vi "Choose_Plug_In_to_Run.vi"(2 "setup":T1, 3 "Show Panel?":bool, 4 "Setup String In":string) -> (1 "Setup String Out":string)   [LabVIEW 2022 SP3]
uses:
  Anemometry Sub Vis/Controls/ok_button.ctl
  Anemometry Sub Vis/Controls/Setup.ctl
  Anemometry Sub Vis/Controls/Post_Process.ctl
  Anemometry Sub Vis/Globals/Meas_global.vi
  Anemometry Sub Vis/Globals/Dynamic_call_global.ph.vi
panel:
  in  "Deselect Pre Analysis Plugins":bool
  in  "Pre_Analysis_Plugins":i32[](listbox)
  in  "Deselect Final":bool
  in  "Deselect per block":bool
  in  "Deselect Initial":bool
  in  "Override Post Process Plugins Setup":bool
  in  "OK Button":T2
  in  "Final Plug In":i32[](listbox)
  in  "Per Block Plug ins":i32[](listbox)
  in  "Initial Plug Ins":i32[](listbox)
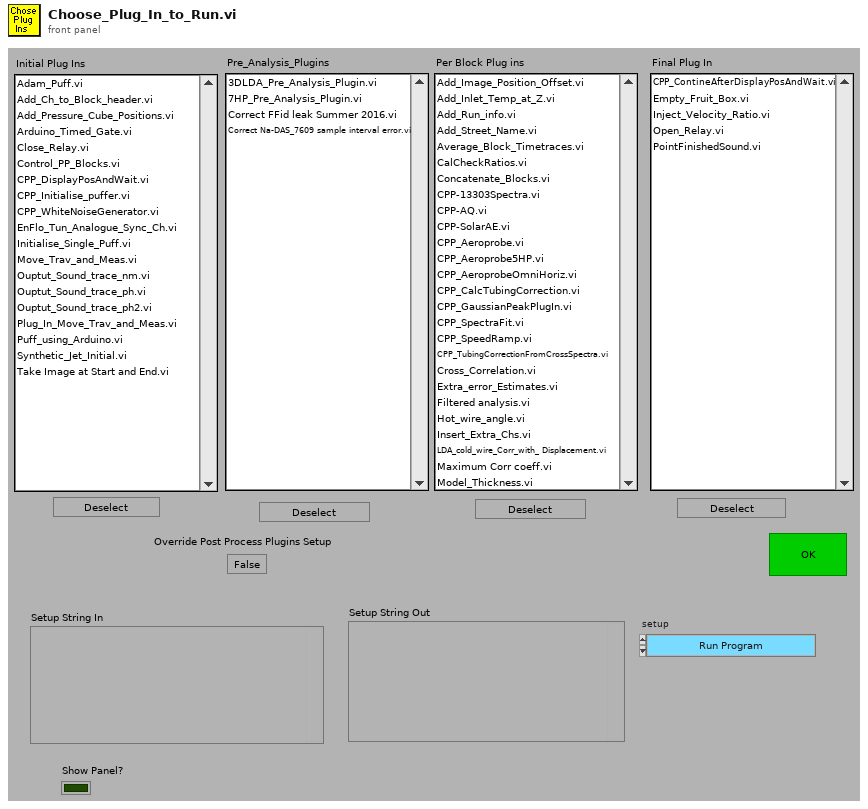
[diagram p1: front panel]
types:
  T1 = typedef "Setup.ctl" = enum16{"Run Program", "Show Setup", "Save Current Setup", "Setup Front Panel"}
  T2 = typedef "ok_button.ctl" = bool
  T3 = typedef "Post_Process.ctl" = enum16{"Take New Data", "Post Process Raw Data File"}
  T4 = enum32{"Invalid", "Standard", "Closed", "Hidden", "Minimized", "Maximized"}
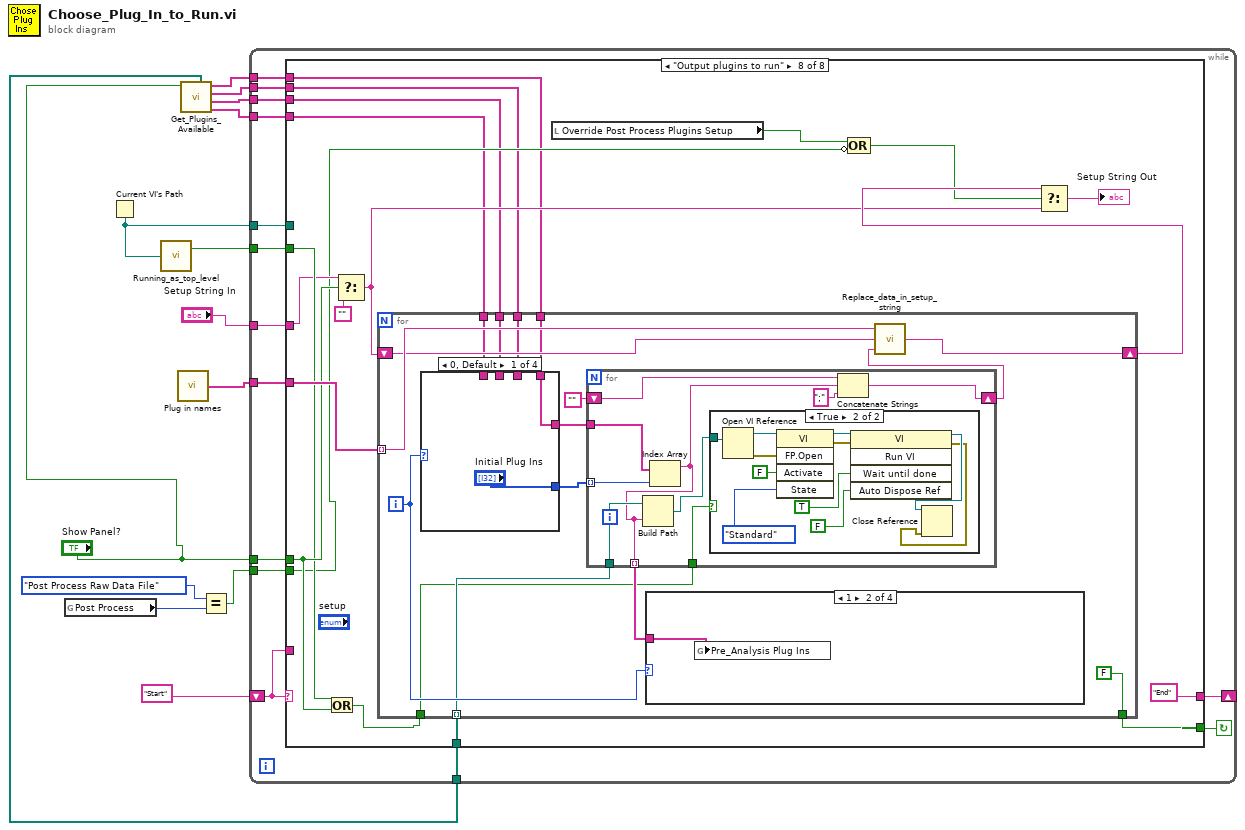
[diagram p0: block diagram]
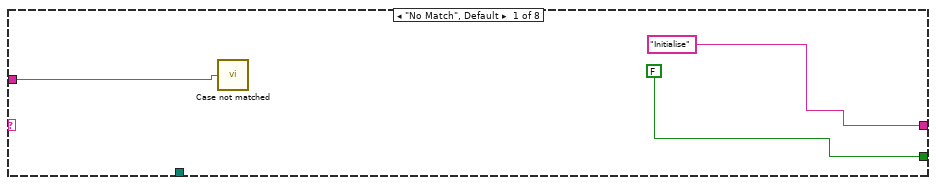
[diagram p2: hidden frame]
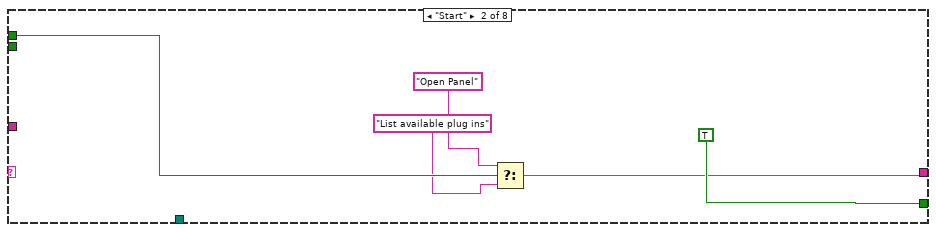
[diagram p3: hidden frame]
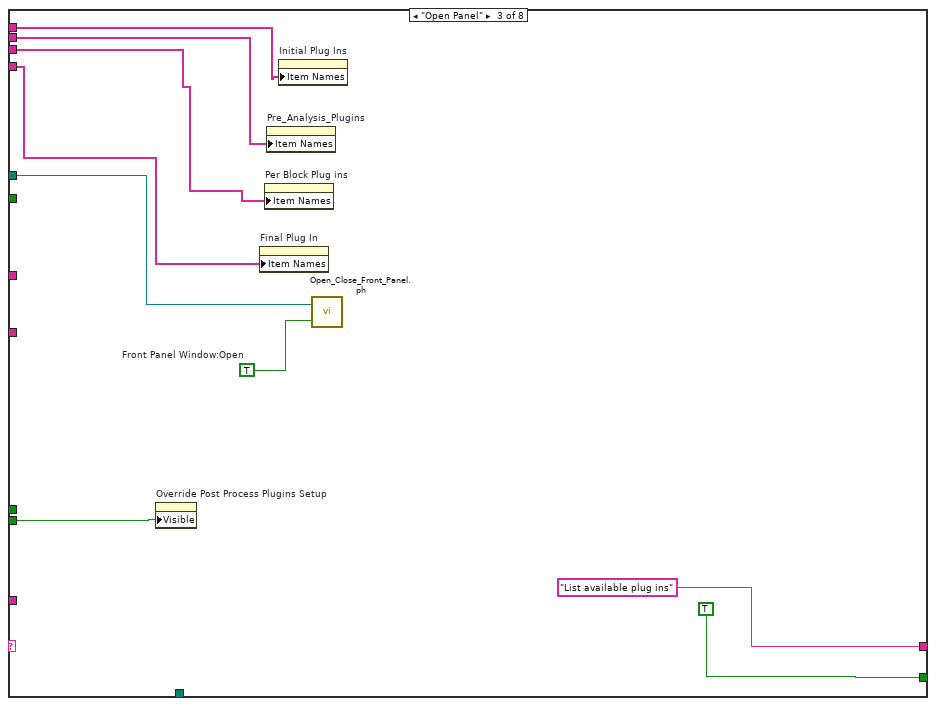
[diagram p4: hidden frame]
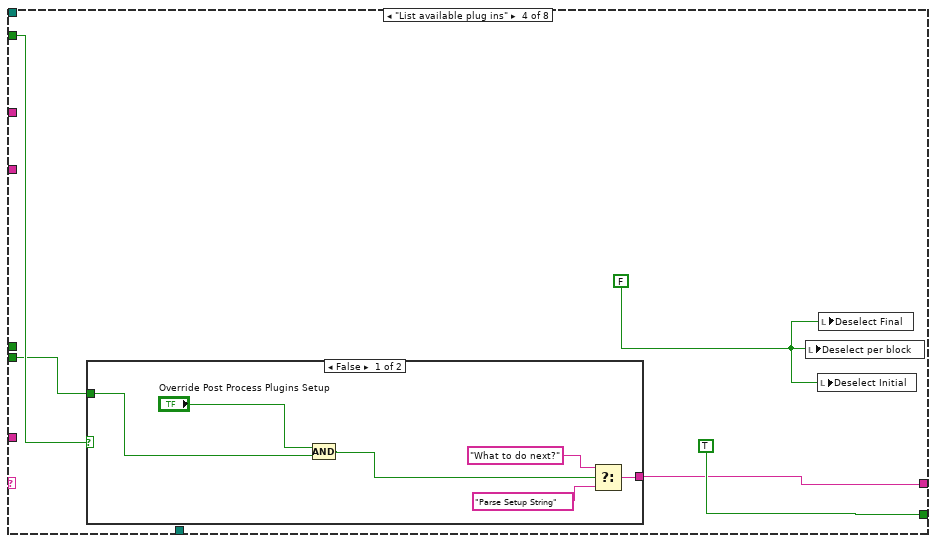
[diagram p5: hidden frame]
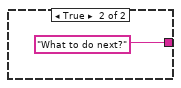
[diagram p6: hidden frame]
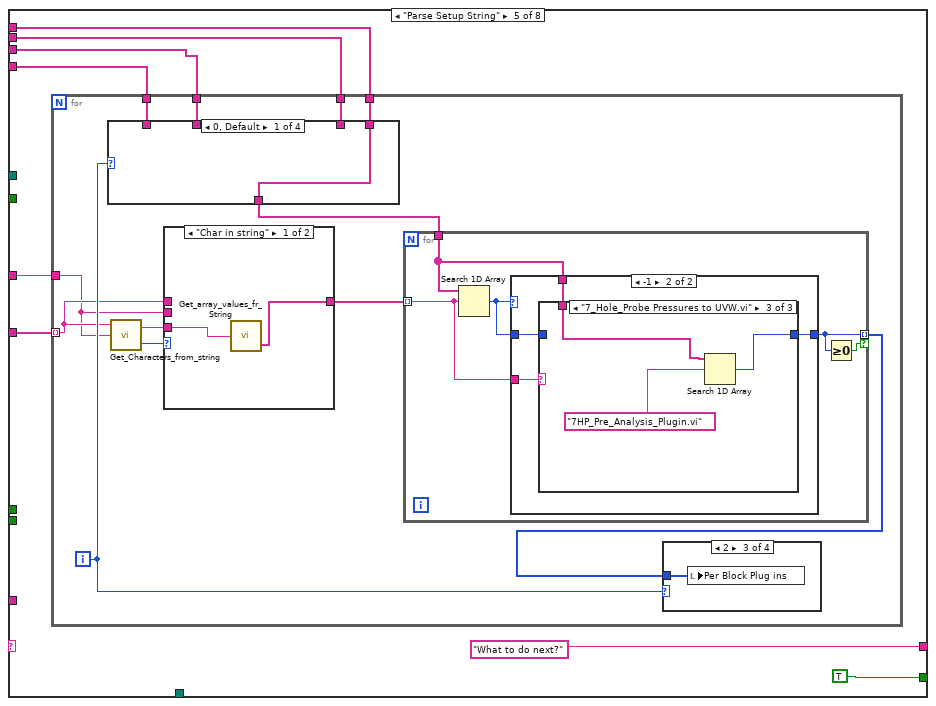
[diagram p7: hidden frame]
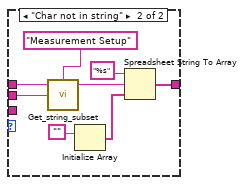
[diagram p8: hidden frame]
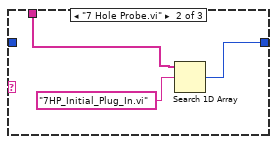
[diagram p11: hidden frame]
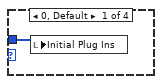
[diagram p15: hidden frame]
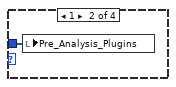
[diagram p16: hidden frame]
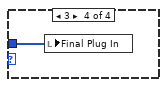
[diagram p17: hidden frame]
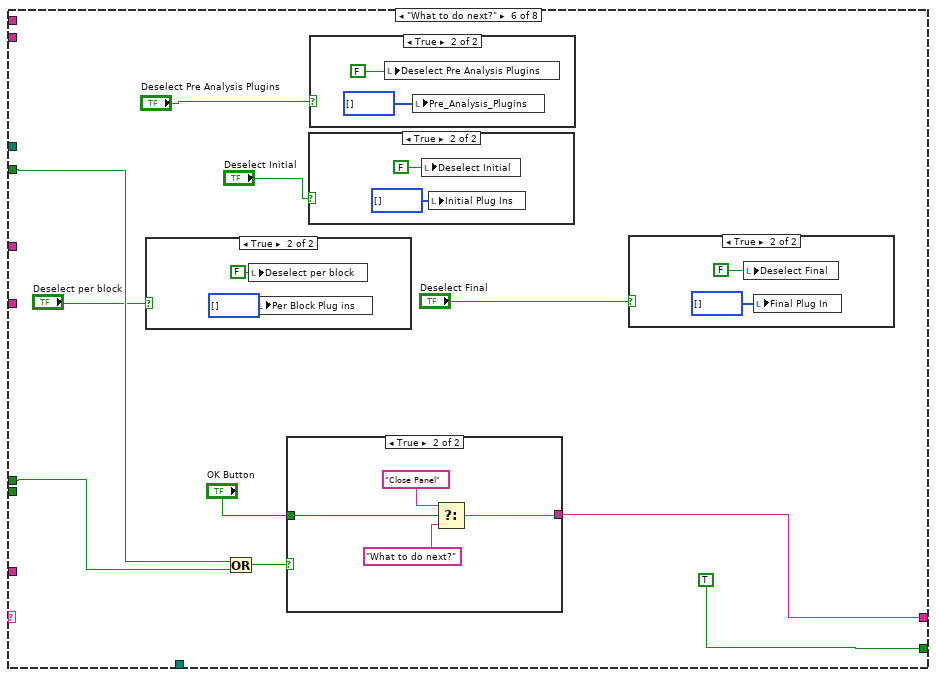
[diagram p18: hidden frame]
diagram:
  n1 = global read "Meas_global.vi" "Post Process"() -> (w9:T3)
  n2 = Current VI's Path() -> (path=w11:path)
  n3 = call "Running_as_top_level.vi"("Vi path name"=w11) -> ("Top Level"=w12:bool)  [unwired: 1 out]
  n4 = call "Plug in names.vi"() -> ("Array"=w1:string[])  [unwired: 1 in]
  n5 = call "Get_Plugins_Available.vi"("Reload Available Plugins"="Show Panel?") -> ("Final"=w4:string[], "Per Block"=w5:string[], "Pre-Analysis"=w6:string[], "Initial"=w7:string[], "Directories"=w3:path[])  [unwired: 6 in]
  n6 = Equal?(x=Post_Process."Post Process Raw Data File" ("Post Process"), y=w9) -> (x = y?=w8:bool)
  n7 = while {
    shift-left: "Start" -> [w26]
    shift-right: [w27] -> _
    tunnel: w1 -> [w25]
    tunnel: "Show Panel?" -> [w24]
    tunnel: "Setup String In" -> [w23]
    tunnel: w12 -> [w22]
    tunnel: w11 -> [w21]
    tunnel: w8 -> [w20]
    tunnel: w7 -> [w19]
    tunnel: w6 -> [w18]
    tunnel: w5 -> [w17]
    tunnel: w4 -> [w16]
    tunnel: w3 -> [w15]
    stop <- w28 continue-if-true
    n8 = case shown="\"Output plugins to run\"" w26 {
      tunnel: [FALSE TRUE TRUE TRUE TRUE TRUE TRUE w151] -> w28
      tunnel: ["Initialise" w32 "List available plug ins" ("f") w49 "What to do next?" ("t") w120 "Output plugins to run" ("f") "End"] -> w27
      tunnel: w26 -> [w29 _ _ _ _ _ _ _]
      tunnel: w25 -> [_ _ _ _ w64 _ _ w169]
      tunnel: w24 -> [_ w34 _ _ _ w119 _ w167]
      tunnel: w23 -> [_ _ _ _ w63 _ _ w161]
      tunnel: w22 -> [_ _ _ w48 _ w118 w138 w166]
      tunnel: w21 -> [_ _ w42 _ _ _ _ _]
      tunnel: w20 -> [_ _ w41 w46 _ _ w136 w157]
      tunnel: w19 -> [_ _ w37 _ w61 _ _ w156]
      tunnel: w18 -> [_ _ w38 _ w60 _ _ w155]
      tunnel: w17 -> [_ _ w39 _ w59 _ _ w154]
      tunnel: w16 -> [_ _ w40 _ w58 _ _ w153]
      tunnel: w15 -> [_ _ _ _ _ _ _ w152]
      frame "No Match", Default {
        n9 = call "Case not matched.vi"("Case Name not Matched"=w29) -> ()
      }
      frame "Start" {
        n10 = Select(t="Open Panel", s=w34, f="List available plug ins") -> (s? t:f=w32:string)
      }
      frame "Open Panel" {
        w44 = TRUE  # Front Panel Window:Open
        n11 = property on="Override Post Process Plugins Setup" class="Bool (strict)"("Visible"=w41) -> ()  [unwired: 2 in, 2 out]
        n12 = property on="Final Plug In" class="LstBox (strict)"("Item Names"=w40) -> ()  [unwired: 2 in, 2 out]
        n13 = property on="Per Block Plug ins" class="LstBox (strict)"("Item Names"=w39) -> ()  [unwired: 2 in, 2 out]
        n14 = property on="Pre_Analysis_Plugins" class="LstBox (strict)"("Item Names"=w38) -> ()  [unwired: 2 in, 2 out]
        n15 = property on="Initial Plug Ins" class="LstBox (strict)"("Item Names"=w37) -> ()  [unwired: 2 in, 2 out]
        n16 = call "Open_Close_Front_Panel.ph.vi"("openWindow (T)"=w44, "VI path"=w42) -> ()  [unwired: 1 in, 1 out]
      }
      frame "List available plug ins" {
        w47 = FALSE
        n17 = case shown="False" w48 {
          tunnel: [w52 "What to do next?"] -> w49
          tunnel: w46 -> [w51 _]
          frame False {
            n18 = Compound Arithmetic op=AND("Override Post Process Plugins Setup", w51) -> (w55:bool)
            n19 = Select(t="What to do next?", s=w55, f="Parse Setup String") -> (s? t:f=w52:string)
          }
          frame True {
          }
        }
        n20 = local write "Deselect per block"(w47) -> ()
        n21 = local write "Deselect Initial"(w47) -> ()
        n22 = local write "Deselect Final"(w47) -> ()
      }
      frame "Parse Setup String" {
        n23 = for {
          tunnel: w64 -> [w75] mode=indexing
          tunnel: w63 -> [w74]
          tunnel: w61 -> [w69]
          tunnel: w60 -> [w68]
          tunnel: w59 -> [w67]
          tunnel: w58 -> [w66]
          i -> [w77]
          n24 = case shown="0, Default" w77 {
            tunnel: [w105 w106 w107 w108] -> w76
            tunnel: w69 -> [w105 _ _ _]
            tunnel: w68 -> [_ w106 _ _]
            tunnel: w67 -> [_ _ w107 _]
            tunnel: w66 -> [_ _ _ w108]
            frame 0, Default {
            }
            frame 1 {
            }
            frame 2 {
            }
            frame 3 {
            }
          }
          n25 = call "Get_Characters_from_string.vi"("Input string"=w74, "Variable name"=w75) -> ("Status"=w72:enum16{"Char in string", "Char not in string"}, "Value"=w71:string)  [unwired: 1 in]
          n26 = case shown="\"Char in string\"" w72 {
            tunnel: w75 -> [_ w87]
            tunnel: w74 -> [_ w86]
            tunnel: [w78 w82] -> w73
            tunnel: w71 -> [w79 _]
            frame "Char in string" {
              n27 = call "Get_array_values_fr_String.vi"("String Value"=w79) -> ("String array"=w78:string[])  [unwired: 1 out]
            }
            frame "Char not in string" {
              n28 = call "Get_string_subset.vi"("String Name"="Measurement Setup", "String to split"=w86, "File Label"=w87) -> ("Output string"=w81:string)  [unwired: 1 in, 1 out]
              n29 = Initialize Array("") -> (w85:string[])  [unwired: 1 out]
              n30 = Spreadsheet String To Array(format string="%s", spreadsheet string=w81, array type (2D Dbl)=w85) -> (array=w82:string[])  [unwired: 1 out]
            }
          }
          n31 = for {
            tunnel: w76 -> [w90]
            tunnel: w73 -> [w91] mode=indexing
            tunnel: [w89] -> w70 mode=indexing if=w88
            n32 = Search 1D Array(1D array=w90, element=w91) -> (index of element=w92:i32)  [unwired: 1 out]
            n33 = case shown="-1" w92 {
              tunnel: w92 -> [w93 w94]
              tunnel: w91 -> [_ w97]
              tunnel: w90 -> [_ w96]
              tunnel: [w93 w95] -> w89
              frame Default {
              }
              frame -1 {
                n34 = case shown="\"7_Hole_Probe Pressures to UVW.vi\"" w97 {
                  tunnel: w96 -> [_ w100 w103]
                  tunnel: [w98 w99 w102] -> w95
                  tunnel: w94 -> [w98 _ _]
                  frame Default {
                  }
                  frame "7 Hole Probe.vi" {
                    n35 = Search 1D Array(1D array=w100, element="7HP_Initial_Plug_In.vi") -> (index of element=w99:i32)  [unwired: 1 out]
                  }
                  frame "7_Hole_Probe Pressures to UVW.vi" {
                    n36 = Search 1D Array(1D array=w103, element="7HP_Pre_Analysis_Plugin.vi") -> (index of element=w102:i32)  [unwired: 1 out]
                  }
                }
              }
            }
            n37 = Greater Or Equal To 0?(x=w89) -> (x >= 0?=w88:bool)
          }
          n38 = case shown="2" w77 {
            tunnel: w70 -> [w109 w110 w111 w112]
            frame 0, Default {
              n39 = local write "Initial Plug Ins"(w109) -> ()
            }
            frame 1 {
              n40 = local write "Pre_Analysis_Plugins"(w110) -> ()
            }
            frame 2 {
              n41 = local write "Per Block Plug ins"(w111) -> ()
            }
            frame 3 {
              n42 = local write "Final Plug In"(w112) -> ()
            }
          }
        }
      }
      frame "What to do next?" {
        n43 = case shown="True" "Deselect per block" {
          frame False {
          }
          frame True {
            n44 = local write "Deselect per block"(FALSE ("Deselect Initial")) -> ()
            n45 = local write "Per Block Plug ins"(i32[] [] ("Initial Plug Ins")) -> ()
          }
        }
        n46 = Or(x=w118, y=w119) -> (x .or. y?=w117:bool)
        n47 = case shown="True" w117 {
          tunnel: "OK Button" -> [_ w135]
          tunnel: ["Output plugins to run" w132] -> w120
          frame False {
          }
          frame True {
            n48 = Select(t="Close Panel", s=w135, f="What to do next?") -> (s? t:f=w132:string)
          }
        }
        n49 = case shown="True" "Deselect Initial" {
          frame False {
          }
          frame True {
            n50 = local write "Deselect Initial"(FALSE ("Deselect Initial")) -> ()
            n51 = local write "Initial Plug Ins"(i32[] [] ("Initial Plug Ins")) -> ()
          }
        }
        n52 = case shown="True" "Deselect Pre Analysis Plugins" {
          frame False {
          }
          frame True {
            n53 = local write "Deselect Pre Analysis Plugins"(FALSE ("Deselect Initial")) -> ()
            n54 = local write "Pre_Analysis_Plugins"(i32[] [] ("Initial Plug Ins")) -> ()
          }
        }
        n55 = case shown="True" "Deselect Final" {
          frame False {
          }
          frame True {
            n56 = local write "Deselect Final"(FALSE ("Deselect Initial")) -> ()
            n57 = local write "Final Plug In"(i32[] [] ("Initial Plug Ins")) -> ()
          }
        }
      }
      frame "Close Panel" {
        n58 = case shown="False" w138 {
          tunnel: w136 -> [w140 _]
          frame False {
            n59 = stacked-sequence {
              tunnel: w140 -> [w141 _]
              frame #0 {
                n60 = local read "Override Post Process Plugins Setup"() -> (w143:bool)
                n61 = Compound Arithmetic op=AND(w141, invert w143) -> (w142:bool)
                n62 = case shown="True" w142 {
                  frame False {
                  }
                  frame True {
                    n63 = Two Button Dialog(message="Do you want to override the plugins setup whilst post processing?", 1:"No" ("F button name (\"Cancel\")"), 2:"Yes" ("T button name (\"OK\")")) -> (T button?=w146:bool)
                    n64 = case shown="True" w146 {
                      tunnel: w146 -> [_ w148]
                      frame False {
                      }
                      frame True {
                        n65 = local write "Override Post Process Plugins Setup"(w148) -> ()
                      }
                    }
                  }
                }
              }
              frame #1 {
                w150 = FALSE  # Front Panel Window:Open
                n66 = Current VI's Path() -> (path=w149:path)
                n67 = call "Open_Close_Front_Panel.ph.vi"("openWindow (T)"=w150, "VI path"=w149) -> ()  [unwired: 1 in, 1 out]
              }
            }
          }
          frame True {
          }
        }
      }
      frame "Output plugins to run" {
        n68 = Or(x=w166, y=w167) -> (x .or. y?=w165:bool)
        n69 = Select(t=w161, s=w167, f="") -> (s? t:f=w160:string)
        n70 = for {
          shift-right: [w179] -> w163
          shift-left: w160 -> [w177]
          tunnel: w152 -> [w183] mode=indexing
          tunnel: w169 -> [w178] mode=indexing
          tunnel: w165 -> [w181]
          tunnel: w156 -> [w174]
          tunnel: w155 -> [w173]
          tunnel: w154 -> [w172]
          tunnel: w153 -> [w171]
          tunnel: [FALSE] -> w151
          i -> [w184]
          n71 = case shown="0, Default" w184 {
            tunnel: ["Initial Plug Ins" "Pre_Analysis_Plugins" "Per Block Plug ins" "Final Plug In"] -> w185
            tunnel: [w195 w197 w199 w201] -> w180
            tunnel: w174 -> [w195 _ _ _]
            tunnel: w173 -> [_ w197 _ _]
            tunnel: w172 -> [_ _ w199 _]
            tunnel: w171 -> [_ _ _ w201]
            frame 0, Default {
            }
            frame 1 {
            }
            frame 2 {
            }
            frame 3 {
            }
          }
          n72 = for {
            tunnel: w185 -> [w211] mode=indexing
            tunnel: w183 -> [w210]
            tunnel: [w204] -> w182 mode=indexing
            tunnel: w181 -> [w209]
            tunnel: w180 -> [w207]
            shift-right: [w205] -> w175
            shift-left: "" -> [w206]
            n73 = Index Array(array=w207, index=w211) -> (element=w204:string)
            n74 = Build Path(base path=w210, name or relative path=w204) -> (appended path=w208:path)
            n75 = case shown="True" w209 {
              tunnel: w208 -> [_ w222]
              frame False {
              }
              frame True {
                n76 = Open VI Reference(vi path=w222) -> (vi reference=w219:refnum<vi>, error out=w218:errorcluster)  [unwired: 1 in, 4 out]
                n77 = invoke class="VI" method="FP.Open"(reference=w219, error in=w218, "Activate"=FALSE ("Activate?"), "State"=T4."Standard") -> (reference out=w217:refnum<vi>, error out=w216:errorcluster)  [unwired: 1 in, 3 out]
                n78 = invoke class="VI" method="Run VI"(reference=w217, error in=w216, "Wait until done"=TRUE, "Auto Dispose Ref"=FALSE) -> (reference out=w215:refnum<vi>, error out=w214:errorcluster)  [unwired: 1 in, 3 out]
                n79 = Close Reference(reference=w215, error in (no error)=w214) -> ()  [unwired: 1 out]
              }
            }
            n80 = Concatenate Strings(w206, w204, ";" ("string")) -> (w205:string)
          }
          n81 = case shown="1" w184 {
            tunnel: w182 -> [w186 w187 w189 w194]
            frame 0, Default {
              n82 = global write "Dynamic_call_global.ph.vi" "Initial Plug Ins"(w186) -> ()
            }
            frame 1 {
              n83 = global write "Dynamic_call_global.ph.vi" "Pre_Analysis Plug Ins"(w187) -> ()
            }
            frame 2 {
              n84 = for {
                tunnel: w189 -> [w191] mode=indexing
                tunnel: [w190] -> w188 mode=indexing
                n85 = case shown="\"Puff_release2_chs.vi\"" w191 {
                  selector: w191 -> [_ w193]
                  tunnel: ["Puff_Dose.vi" w193] -> w190
                  frame "Puff_release2_chs.vi" {
                  }
                  frame Default {
                  }
                }
              }
              n86 = global write "Dynamic_call_global.ph.vi" "Per Block Plug Ins"(w188) -> ()
            }
            frame 3 {
              n87 = global write "Dynamic_call_global.ph.vi" "Final Plug Ins"(w194) -> ()
            }
          }
          n88 = call "Replace_data_in_setup_string.vi"("New data string"=w175, "Input string"=w177, "Variable name"=w178) -> ("Appended string"=w179:string)
        }
        n89 = local read "Override Post Process Plugins Setup"() -> (w159:bool)
        n90 = Compound Arithmetic op=OR(w159, invert w157) -> (w158:bool)
        n91 = Select(t=w163, s=w158, f=w160) -> (s? t:f=→"Setup String Out":string)
      }
    }
  }
